vi "FTW-CodeGen-Bounds.vi"(0 "State In":T1, 5 "XRef":refnum<vi>) -> (4 "Bounds":cluster{"Width":i32, "Height":i32})   [LabVIEW 2014, in "FTW-Sync-Synchronizer.xnode"]
uses:
  FTW-Sync-Synchronizer.xnode
  FTW-CodeGen-State.ctl
panel:
  # "Inputs"
  # "Outputs"
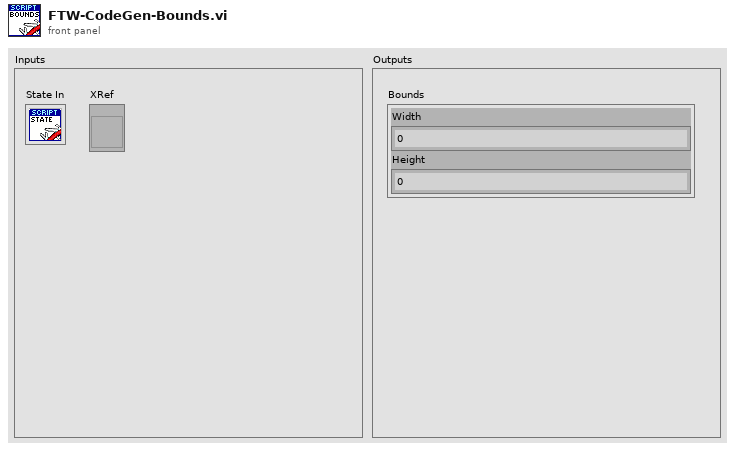
[diagram p1: front panel]
types:
  T1 = typedef "FTW-Sync-Synchronizer.xnode/FTW-CodeGen-State.ctl" = cluster{"InputTerminals":cluster{"Wired?":bool, "ID":string, "DataName":string, "DataColor":u32, "Type":variant}[], "EnableTiming?":bool}
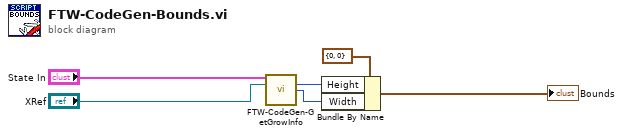
[diagram p0: block diagram]
diagram:
  n1 = call "FTW-CodeGen-GetGrowInfo.vi"("State In"="State In", "XRef"="XRef") -> ("Current Height"=w2:i32, "Width"=w1:i32)  [unwired: 5 in, 7 out]
  n2 = Bundle By Name(cluster=cluster{"Width":i32, "Height":i32} {"Width"=0, "Height"=0} ("Bounds"), "Height"=w2, "Width"=w1) -> (→"Bounds":cluster{"Width":i32, "Height":i32})
